vi "Teleop.vi"(10 "Match Info":T1={"Autonomous Elapsed Seconds"=0.0, "TeleOp Elapsed Seconds"=0.0, "Disabled Elapsed Seconds"=0.0, "Visited Autonomous"=FALSE, "Visited TeleOp"=FALSE, "Visited Disabled"=FALSE, "Autonomous Settings"={"Autonomous Style"=enum."Independent", "VI Refnum"=refnum}}, 11 "Call Context":T2) -> ()   [LabVIEW 2020]
doc: "This VI is called for each TeleOp packet received from the DS where the robot is not disabled. It is often used to read from the joysticks and update I/O or to update setpoints for timed control loops. It should complete and return within 20 milliseconds or it may miss DS packets."
uses:
  <vilib>/Rock Robotics/WPI/DriverStation/WPI_DriverStationDerivedRobotMode.ctl
  <vilib>/Rock Robotics/WPI/DriverStation/WPI_DriverStationMatch Info.ctl
panel:
  out "% voltage":dbl
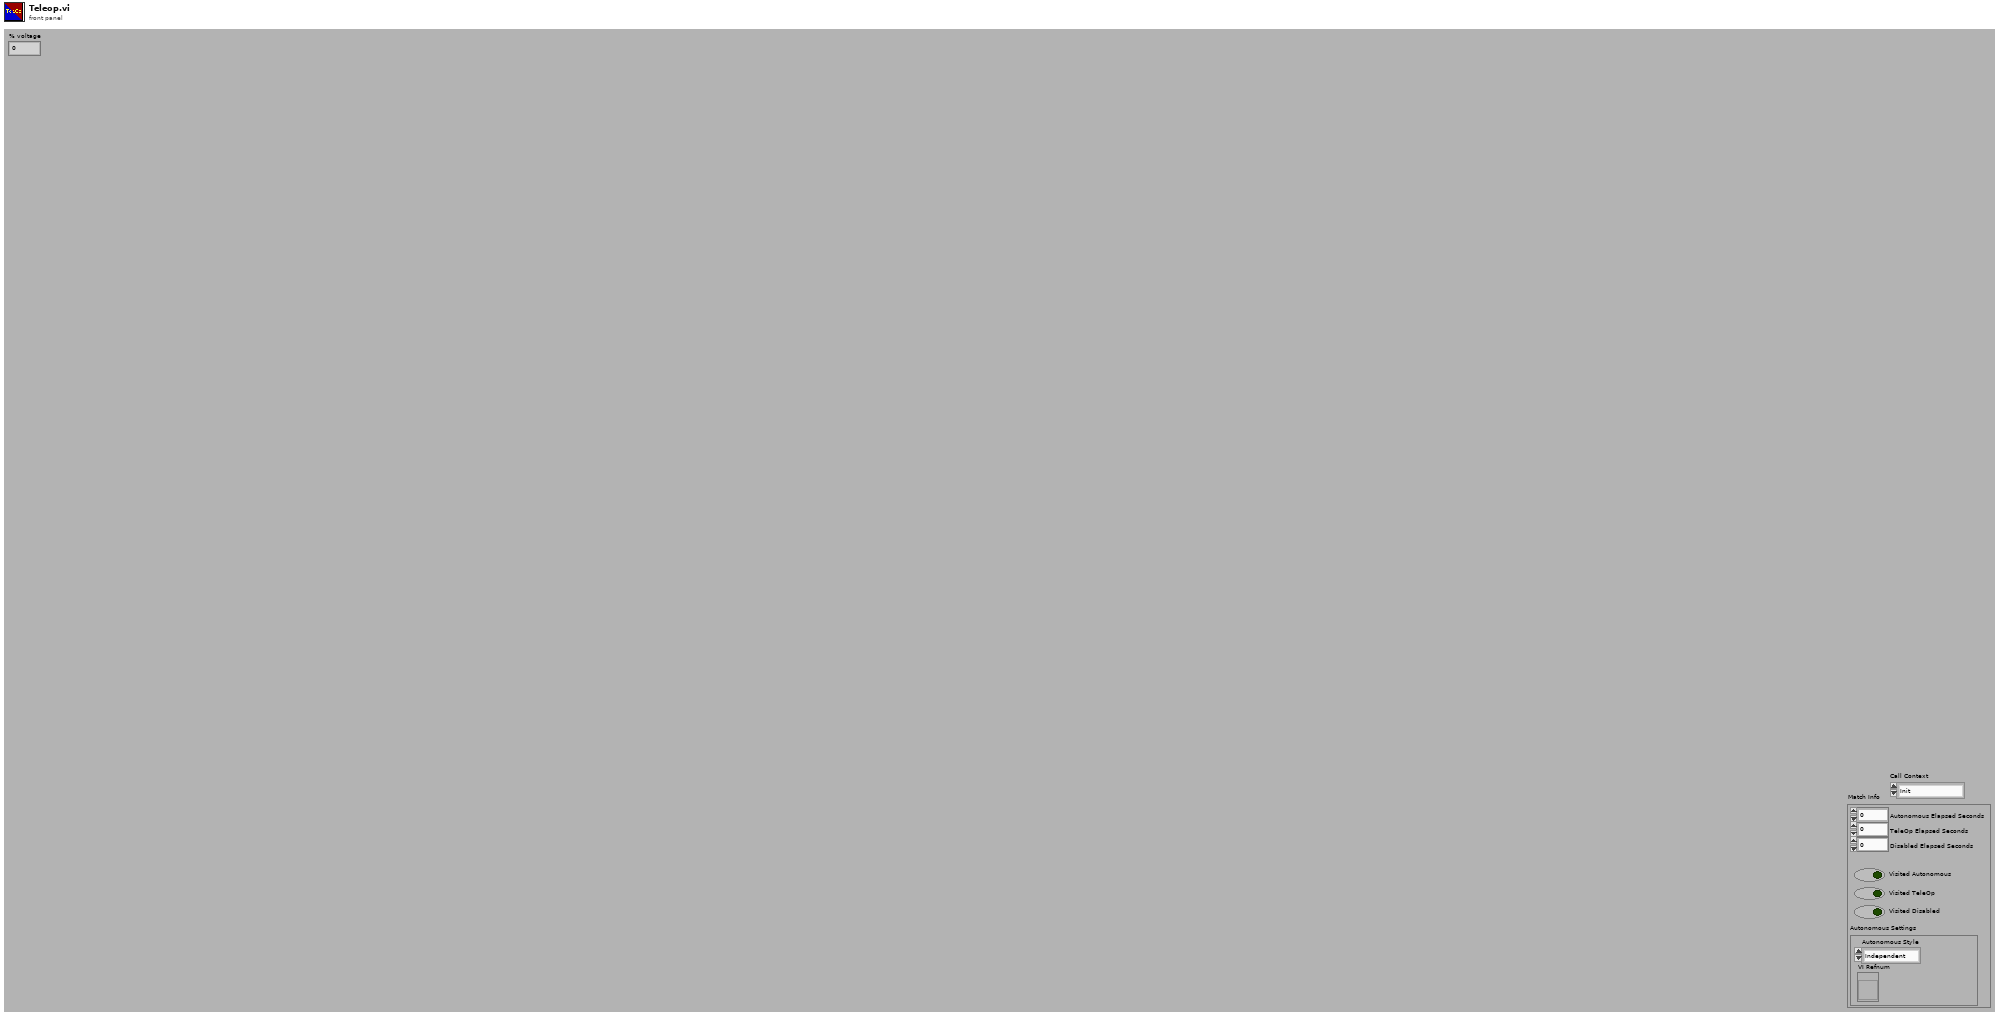
[diagram p1: front panel]
types:
  T1 = typedef "WPI_DriverStationMatch Info.ctl" = cluster{"Autonomous Elapsed Seconds":dbl, "TeleOp Elapsed Seconds":dbl, "Disabled Elapsed Seconds":dbl, "Visited Autonomous":bool, "Visited TeleOp":bool, "Visited Disabled":bool, "Autonomous Settings":cluster{"Autonomous Style":enum16{"Iterative", "Independent"}, "VI Refnum":refnum<vi>}}
  T2 = typedef "WPI_DriverStationDerivedRobotMode.ctl" = enum16{"Init", "Execute", "Stop"}
  T3 = cluster{"A":bool, "B":bool, "X":bool, "Y":bool, "Left Bumper":bool, "Right Bumper":bool, "View Button":bool, "Menu Button":bool, "Left Joystick Press":bool, "Right Joystick Press":bool, "Left Thumbpad X Axis":dbl, "Left Thumbpad Y Axis":dbl, "Left Trigger":dbl, "Right Trigger":dbl, "Right Thumbpad X Axis":dbl, "Right Thumbpad Y Axis":dbl, "Driver - Trigger":bool, "Driver - Middle Thumb":bool, "Driver - Left Thumb":bool, "Driver - Right Thumb":bool, "Driver - Left Top Left ":bool, "Driver - Left Top Middle":bool, "Driver - Left Top Right":bool, "Driver - Left Bottom Right":bool, "Driver - Left Bottom Middle":bool, "Driver - Left Bottom Left":bool, "Driver - Right Top Right":bool, "Driver - Right Top Middle":bool, "Driver - Right Top Left":bool, "Driver - Right Bottom Left":bool, "Driver - Right Bottom Middle":bool, "Driver - Right Bottom Right":bool, "Driver - X Axis":dbl, "Driver - Y Axis":dbl, "Driver - Z Axis":dbl}
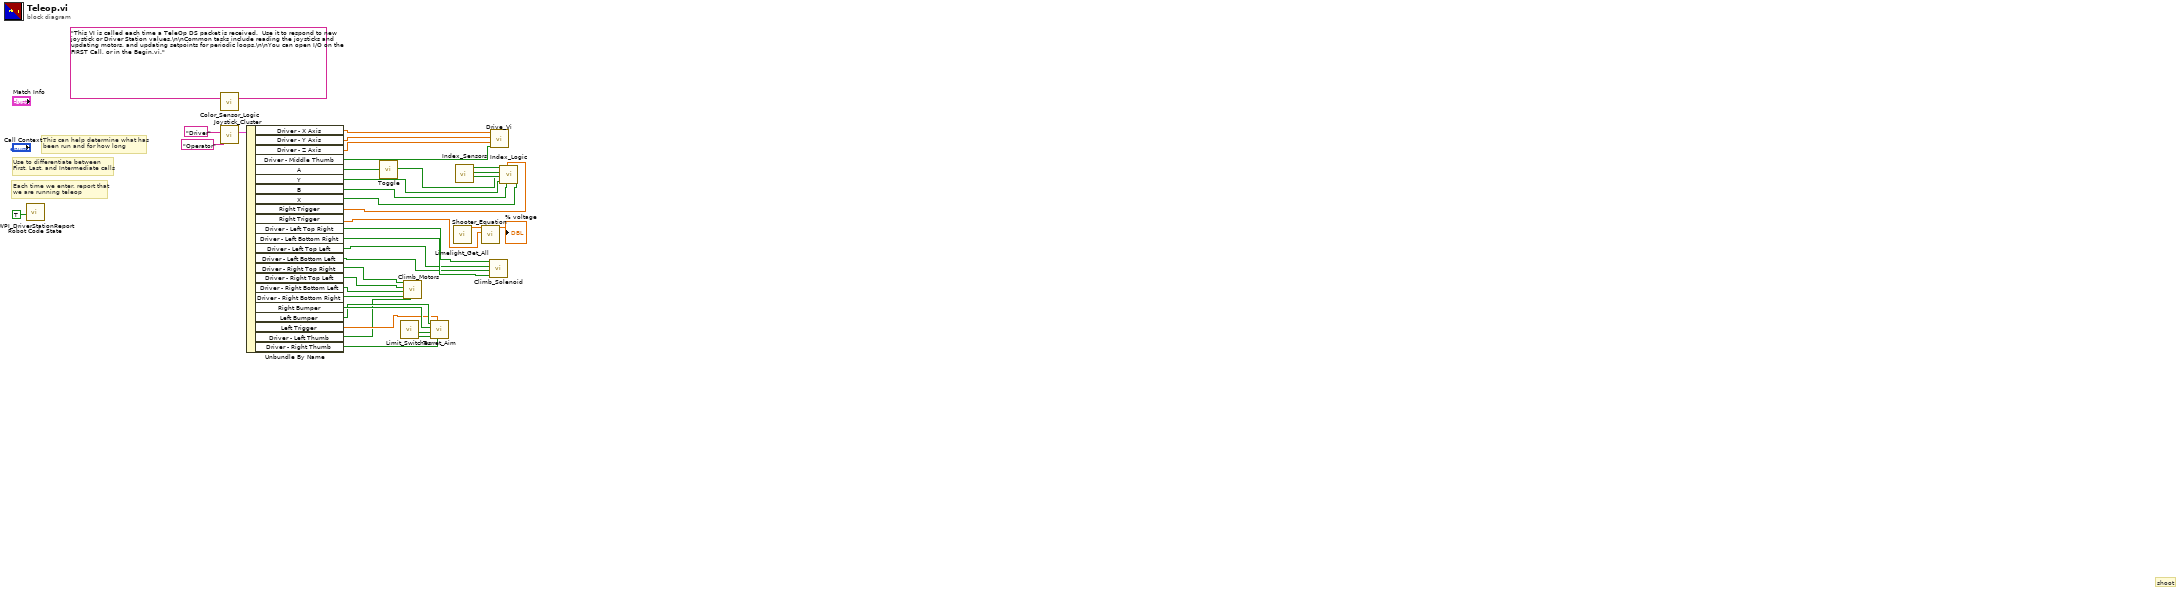
[diagram p0: block diagram]
diagram:
  (unwired) "This VI is called each time a TeleOp DS packet is received.  Use it to respond to new joystick or Driver Station values.\n\nCommon tasks include reading the joysticks and updating motors, and updating setpoints for periodic loops.\n\nYou can open I/O on the FIRST Call, or in the Begin.vi."
  # "shoot"
  # "Each time we enter, report that\nwe are running teleop"
  # "Use to differentiate between\nFirst, Last, and Intermediate calls"
  # "This can help determine what has\nbeen run and for how long"
  n1 = call <vilib>:"WPI_DriverStationReport Robot Code State.vi"("TeleOp"=TRUE ("Autonomous")) -> ()  [unwired: 10 in, 1 out]
  n2 = call "Color_Sensor_Logic.vi"() -> ()  [unwired: 12 in]
  n3 = call "Joystick_Cluster.vi"("Xbox"="Operator", "Thrustmaster"="Driver") -> ("Joystick Output"=w32:T3)  [unwired: 9 in]
  n4 = Unbundle By Name(w32) -> ("Driver - X Axis"=w2:dbl, "Driver - Y Axis"=w3:dbl, "Driver - Z Axis"=w4:dbl, "Driver - Middle Thumb"=w5:bool, "A"=w24:bool, "Y"=w28:bool, "B"=w27:bool, "X"=w26:bool, "Right Trigger"=w25:dbl, "Right Trigger"=w20:dbl, "Driver - Left Top Right"=w19:bool, "Driver - Left Bottom Right"=w18:bool, "Driver - Left Top Left"=w17:bool, "Driver - Left Bottom Left"=w16:bool, "Driver - Right Top Right"=w12:bool, "Driver - Right Top Left"=w13:bool, "Driver - Right Bottom Left"=w14:bool, "Driver - Right Bottom Right"=w15:bool, "Right Bumper"=w9:bool, "Left Bumper"=w8:bool, "Left Trigger"=w7:dbl, "Driver - Left Thumb"=w6:bool, "Driver - Right Thumb"=w1:bool)
  n5 = call "Toggle.vi"("Boolean"=w24) -> ("Boolean Out"=w23:bool)
  n6 = call "Limit_Switches.vi"() -> ("Blue Limit Pressed"=w10:bool, "Orange Limit Pressed"=w11:bool)  [unwired: 10 in]
  n7 = call "Climb_Motors.vi"("Driver - Left Thumb"=w6, "Right Bottom Right"=w15, "Right Bottom Left"=w14, "Right Top Left"=w13, "Right Top Right"=w12) -> ()  [unwired: 7 in]
  n8 = call "Turret_Aim.vi"("Driver Right Thumb"=w1, "Left Trigger"=w7, "Orange Limit Pressed"=w11, "Blue Limit Pressed"=w10, "Right Bumper"=w9, "Left Bumper"=w8) -> ()  [unwired: 6 in]
  n9 = call "Limelight_Get_All.vi"() -> ("Ty"=w22:dbl)  [unwired: 10 in, 1 out]
  n10 = call "Index_Sensors.vi"() -> ("Intake Pressed"=w31:bool, "Reject Pressed"=w30:bool, "Elevate Pressed"=w29:bool)  [unwired: 9 in]
  n11 = call "Shooter_Equation.vi"("Right Trigger"=w20, "Ty"=w22) -> ("% voltage"=→"% voltage":dbl)  [unwired: 9 in]
  n12 = call "Climb_Solenoid.vi"("Left Bottom Right"=w18, "Left Bottom Left"=w16, "Left Top Left"=w17, "Left Top Right"=w19) -> ()  [unwired: 8 in]
  n13 = call "Drive_Vi.vi"("Middle Thumb"=w5, "Z"=w4, "Y"=w3, "X"=w2) -> ()  [unwired: 8 in]
  n14 = call "Index_Logic.vi"("X"=w26, "Intake Pressed"=w31, "B"=w27, "Right Trigger"=w25, "Y"=w28, "A"=w23, "Reject Pressed"=w30, "Elevate Pressed"=w29) -> ()  [unwired: 4 in]
